vi "Custom - Resize FP.vi"(7 "header ref":refnum<vi>, 8 "error in (no error)":errorcluster, 9 "Panel Height":i32, 10 "Panel Width":i32, 11 "VI in":refnum<vi>) -> (0 "error out":errorcluster, 2 "Panel Ref":refnum<vi>, 3 "VI out":refnum<vi>)   [LabVIEW 2021, in "Pop-Up.lvlib" / "Popup.lvclass"]
doc: "customize the front panel by setting up all the positioning based on the size of the panel and delay inputs for now so that the shifting on screen will not be distracting for the user\n\n<b>Code Developed By:</b> +\nDaniel Coons +\nhttps://github.com/danielcoons/tsc-pop-up"
uses:
  Popup.lvclass
  <vilib>/Utility/miscctls.llb/LVPositionTypeDef.ctl
  <vilib>/Utility/miscctls.llb/LVPointTypeDef.ctl
  Popup.lvclass/Popup.ctl
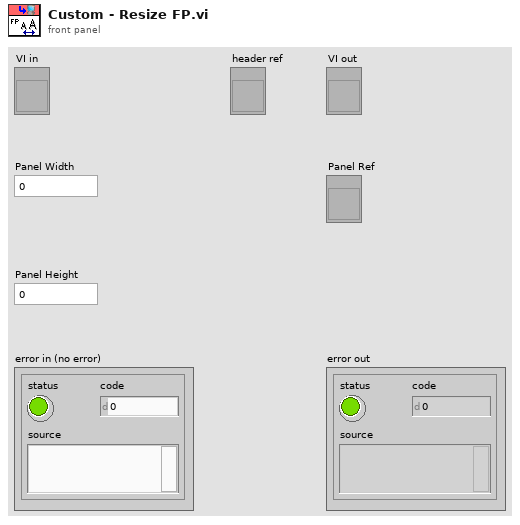
[diagram p1: front panel]
types:
  T1 = typedef "LVPointTypeDef.ctl" = cluster{"Horizontal":i16, "Vertical":i16}
  T2 = typedef "LVPositionTypeDef.ctl" = cluster{"Left":i32, "Top":i32}
  T3 = typedef "LVRectTypeDef.ctl" = cluster{"Left":i16, "Top":i16, "Right":i16, "Bottom":i16}
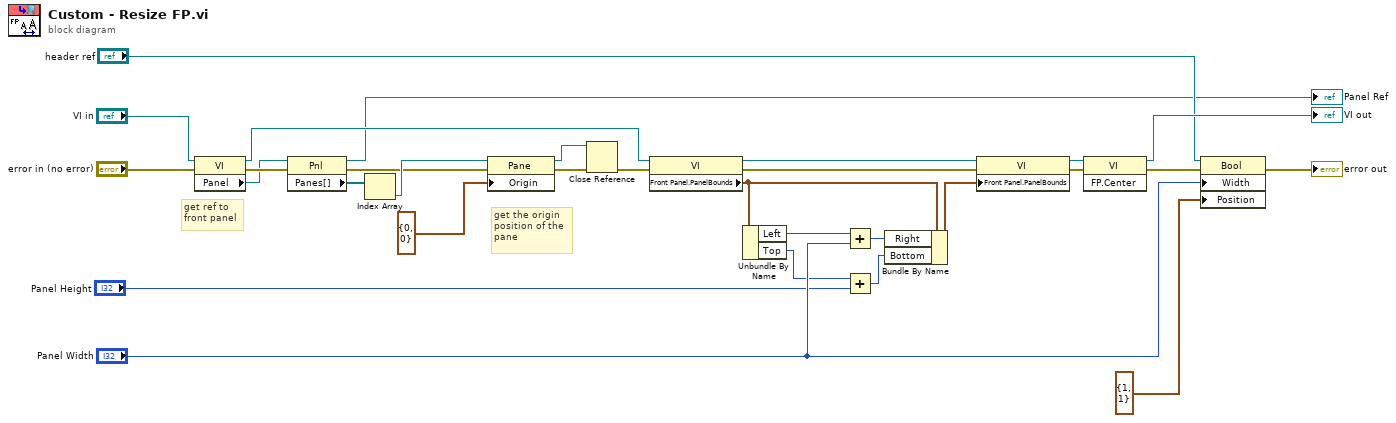
[diagram p0: block diagram]
diagram:
  # "get the origin\nposition of the\npane"
  # "get ref to\nfront panel"
  n1 = property class="VI"(reference="VI in", error in="error in (no error)") -> (reference out=w19:refnum<vi>, error out=w14:errorcluster, "Panel"=w13:refnum<vi>)
  n2 = property class="Pnl"(reference=w13, error in=w14) -> (reference out=→"Panel Ref":refnum<vi>, error out=w16:errorcluster, "Panes[]"=w17:refnum<vi>[])
  n3 = Index Array(array=w17) -> (element=w26:refnum<vi>)  [unwired: 1 in]
  n4 = property class="Pane"(reference=w26, error in=w16, "Origin"=T1 {"Horizontal"=0, "Vertical"=0}) -> (reference out=w28:refnum<vi>, error out=w27:errorcluster)
  n5 = Close Reference(reference=w28, error in (no error)=w27) -> (error out=w3:errorcluster)
  n6 = property class="VI"(reference=w19, error in=w3) -> (reference out=w18:refnum<vi>, error out=w25:errorcluster, "Front Panel.PanelBounds"=w22:T3)
  n7 = Unbundle By Name(w22) -> ("Left"=w30:i16, "Top"=w9:i16)
  n8 = Add(x=w30, y="Panel Width") -> (x+y=w21:i32)
  n9 = Add(x=w9, y="Panel Height") -> (x+y=w7:i32)
  n10 = Bundle By Name(cluster=w22, "Right"=w21, "Bottom"=w7) -> (w15:T3)
  n11 = property class="VI"(reference=w18, error in=w25, "Front Panel.PanelBounds"=w15) -> (reference out=w24:refnum<vi>, error out=w23:errorcluster)
  n12 = invoke class="VI" method="FP.Center"(reference=w24, error in=w23) -> (reference out=→"VI out":refnum<vi>, error out=w20:errorcluster)  [unwired: 1 in, 1 out]
  n13 = property class="Bool"(reference="header ref", error in=w20, "Width"="Panel Width", "Position"=T2 {"Left"=1, "Top"=1}) -> (error out=→"error out":errorcluster)  [unwired: 1 out]
